vi "Create folder if not exist.vi"(8 "Error In":errorcluster, 11 "Folder Path Control":path) -> (0 "Error Out":errorcluster, 3 "Folder Path out":path)   [LabVIEW 2024]
uses:
  <vilib>/Utility/error.llb/Error Cluster From Error Code.vi
  <vilib>/ErrorRing/Error Ring.xnode
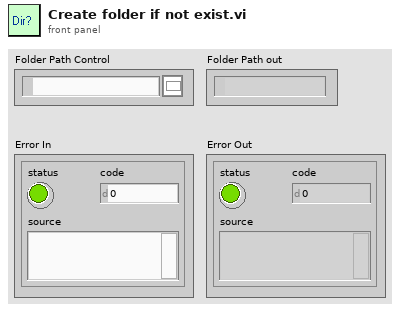
[diagram p1: front panel]
types:
  T1 = cluster{"status":bool, "code":bool, "source":bool}
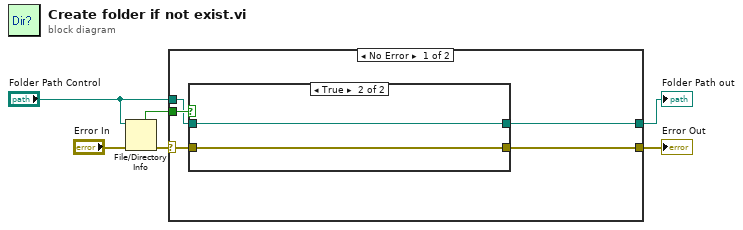
[diagram p0: block diagram]
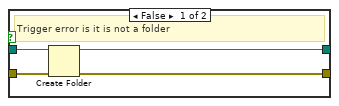
[diagram p2: hidden frame]
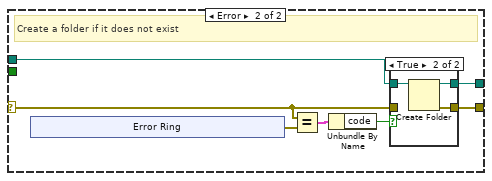
[diagram p3: hidden frame]
diagram:
  n1 = File/Directory Info(path="Folder Path Control", error in="Error In") -> (directory=w6:bool, error out=w1:errorcluster)  [unwired: 5 out]
  n2 = case shown="No Error" w1 {
    selector: w1 -> [w9 w20]
    tunnel: "Folder Path Control" -> [w8 w24]
    tunnel: w6 -> [w11 _]
    tunnel: [w10 w23] -> w4
    tunnel: [w7 w22] -> w2
    frame No Error {
      n3 = case shown="True" w11 {
        tunnel: [w12 w17] -> w10
        tunnel: w9 -> [w13 w17]
        tunnel: w8 -> [w15 w16]
        tunnel: [w14 w16] -> w7
        frame False {
          # "Trigger error is it is not a folder"
          n4 = Create Folder(path (use dialog)=w15, error in=w13) -> (created path=w14:path, error out=w12:errorcluster)  [unwired: 2 out]
        }
        frame True {
        }
      }
    }
    frame Error {
      # "Create a folder if it does not exist"
      n5 = xnode "Error Ring"() -> ("error out"=w21:errorcluster)
      n6 = Equal?(x=w20, y=w21) -> (x = y?=w19:T1)
      n7 = Unbundle By Name(w19) -> ("code"=w18:bool)
      n8 = case shown="True" w18 {
        tunnel: w24 -> [w29 w33]
        tunnel: w20 -> [w30 _]
        tunnel: [w30 w32] -> w23
        tunnel: [w29 w31] -> w22
        frame False {
        }
        frame True {
          n9 = Create Folder(path (use dialog)=w33) -> (created path=w31:path, error out=w32:errorcluster)  [unwired: 1 in, 2 out]
        }
      }
    }
  }
  "Error Out" <- w4
  "Folder Path out" <- w2
